vi "FRCts20_Backend_RequestRoot_POST_return.vi"(7 "Requests":T1, 8 "error in (no error)":errorcluster, 11 "recordset data":variant[][](array[variant])) -> (0 "error out":errorcluster, 3 "data string":string)   [LabVIEW 2014, in "FRCts20_Backend_Engine.lvlib"]
doc: "Returns whether a new request was successfully created & the new request's index"
uses:
  FRCts20_Backend_Engine.lvlib
  FRCts20_Backend_API/Requests.ctl
  FRCts20_Backend_API/Request.ctl
  FRCts20_Backend_API/ApiReturn.ctl
  FRCts20_Backend_API/FRCts20_Backend_API_Status.ctl
  FRCts20_Backend_API/NotesRoot.ctl
  <vilib>/addons/database/_DB Variant To Data/Database Variant To Data.xnode
  FRCts20_Backend_API/FRCts20_Backend_API.lvlib
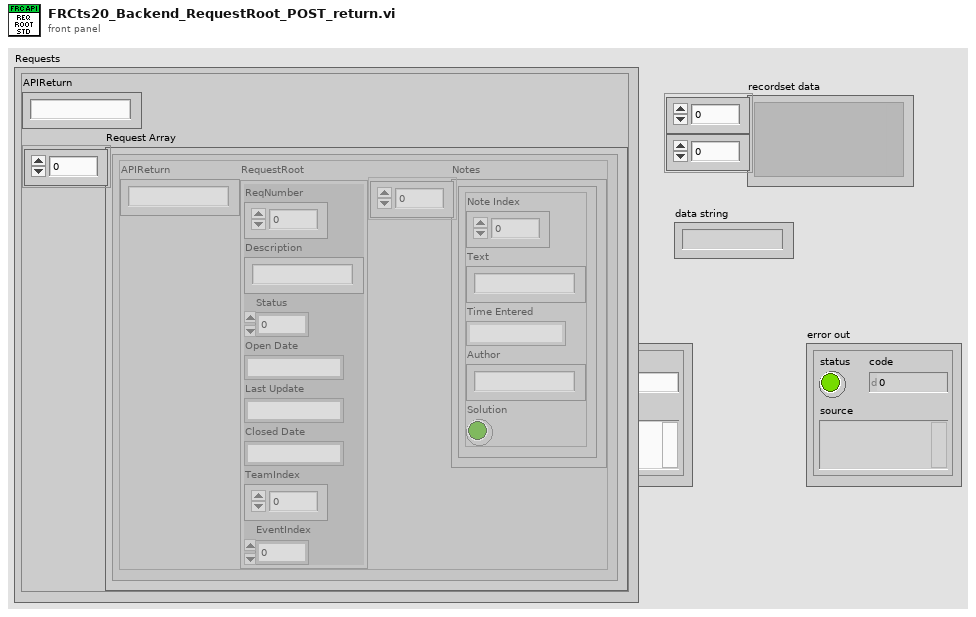
[diagram p1: front panel]
types:
  T1 = typedef "FRCts20_Backend_Engine.lvlib/FRCts20_Backend_API.lvlib/Requests.ctl" = cluster{"APIReturn":string, "Request Array":T2[]}
  T2 = typedef "FRCts20_Backend_Engine.lvlib/FRCts20_Backend_API.lvlib/Request.ctl" = cluster{"APIReturn":T3, "RequestRoot":cluster{"ReqNumber":i32, "Description":string, "Status":T4, "Open Date":string, "Last Update":string, "Closed Date":string, "TeamIndex":i32, "EventIndex":i32}, "Notes":T5}
  T3 = typedef "FRCts20_Backend_Engine.lvlib/FRCts20_Backend_API.lvlib/ApiReturn.ctl" = string
  T4 = typedef "FRCts20_Backend_Engine.lvlib/FRCts20_Backend_API.lvlib/FRCts20_Backend_API_Status.ctl" = i32
  T5 = typedef "FRCts20_Backend_Engine.lvlib/FRCts20_Backend_API.lvlib/NotesRoot.ctl" = cluster{"Note Index":u32, "Text":string, "Time Entered":string, "Author":string, "Solution":bool}[]
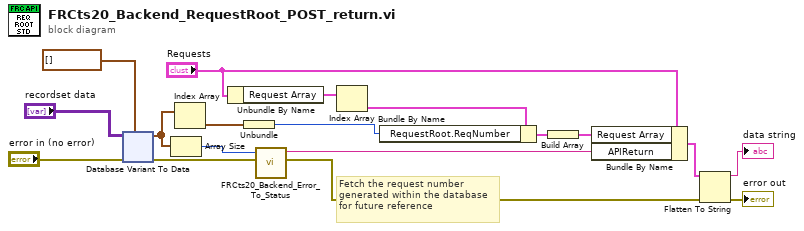
[diagram p0: block diagram]
diagram:
  # "Fetch the request number\ngenerated within the database\nfor future reference"
  n1 = xnode "Database Variant To Data"("database variant"="recordset data", "error in (no error)"="error in (no error)", "type"=cluster{i32}[] []) -> ("data"=w5:cluster{i32}[], "error out"=w17:errorcluster)
  n2 = Array Size(array=w5) -> (size(s)=w4:i32)
  n3 = Index Array(array=w5) -> (element=w13:cluster{i32})  [unwired: 1 in]
  n4 = Unbundle By Name("Requests") -> ("Request Array"=w7:T2[])
  n5 = Unbundle(w13) -> (w3:i32)
  n6 = call "FRCts20_Backend_Error_To_Status.vi"("error in (no error)"=w17, "rows affected"=w4) -> ("error out"=w16:errorcluster, "String"=w18:string)  [unwired: 8 in]
  n7 = Index Array(array=w7) -> (element=w2:T2)  [unwired: 1 in]
  n8 = Bundle By Name(cluster=w2, "RequestRoot.ReqNumber"=w3) -> (w11:T2)
  n9 = Build Array(w11) -> (w1:T2[])
  n10 = Bundle By Name(cluster="Requests", "Request Array"=w1, "APIReturn"=w18) -> (w15:T1)
  n11 = Flatten To String(anything=w15, error in (no error)=w16) -> (data string=→"data string":string, error out=→"error out":errorcluster)  [unwired: 2 in, 1 out]
